vi "Get Source_Voltage Object.vi"   [LabVIEW 2021, in "Source_Voltage.lvclass"]
doc: "This Polymorphic vi returns either a single Source_Voltage object or an array of Source_Voltage objects based on the input pins."
uses:
  Source_Voltage.lvclass
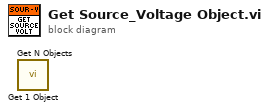
[diagram p0: block diagram]
diagram:
  n1 = call "Get 1 Object.vi"() -> ()  [unwired: 10 in, 2 out]
  n2 = call "Get N Objects.vi"() -> ()  [unwired: 10 in, 2 out]
